vi "2photocell+ledcontrol+sum_cal.vi"() -> ()   [LabVIEW 2016]
uses:
  <vilib>/LabVIEW Interface for Arduino/LabVIEW Interface for Arduino.lvlib
  <vilib>/ptbypt/NI_PtbyPt.lvlib
panel:
  in  "stop":bool
  in  "Tab Control":enum32{"Page 1", "Page 2"}(tab)
  out "LUX":dbl
  out "Voltage":dbl(knob) scale=0.0..5.0
  out "Filtered x":dbl format="%0.2f"
  in  "br_coef":dbl
  in  "thrs low":i32=1
  in  "thrs high":i32=4
  in  "Slide 3":dbl(slide) min=0.0 max=255.0 scale=0.0..255.0
  in  "Slide 2":dbl(slide) min=0.0 max=255.0 scale=0.0..255.0
  in  "Slide":dbl(slide) min=0.0 max=255.0 scale=0.0..255.0
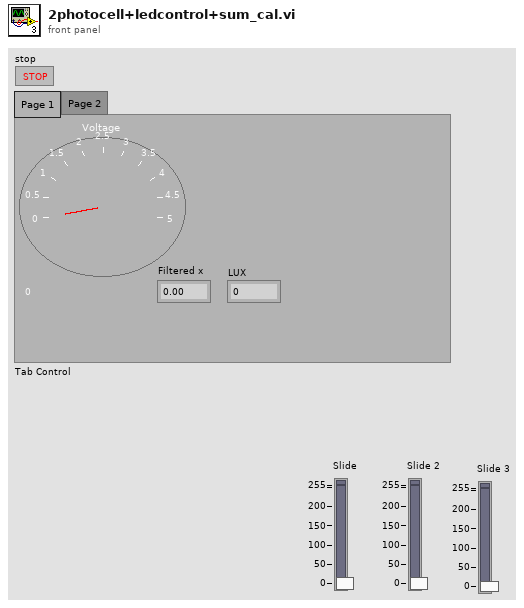
[diagram p1: front panel]
types:
  T1 = typedef "LabVIEW Interface for Arduino.lvlib/Arduino Resource.ctl" = cluster{"VISA resource":refnum<visa-resource-name>, "Board Type":T2, "Connection Type":enum8{"USB / Serial"}, "Bytes Per Packet (15)":u8}
  T2 = typedef "LabVIEW Interface for Arduino.lvlib/Board Type.ctl" = enum16{"Uno", "Dimuelanove w/Atmega 328", "Mega 2560"}
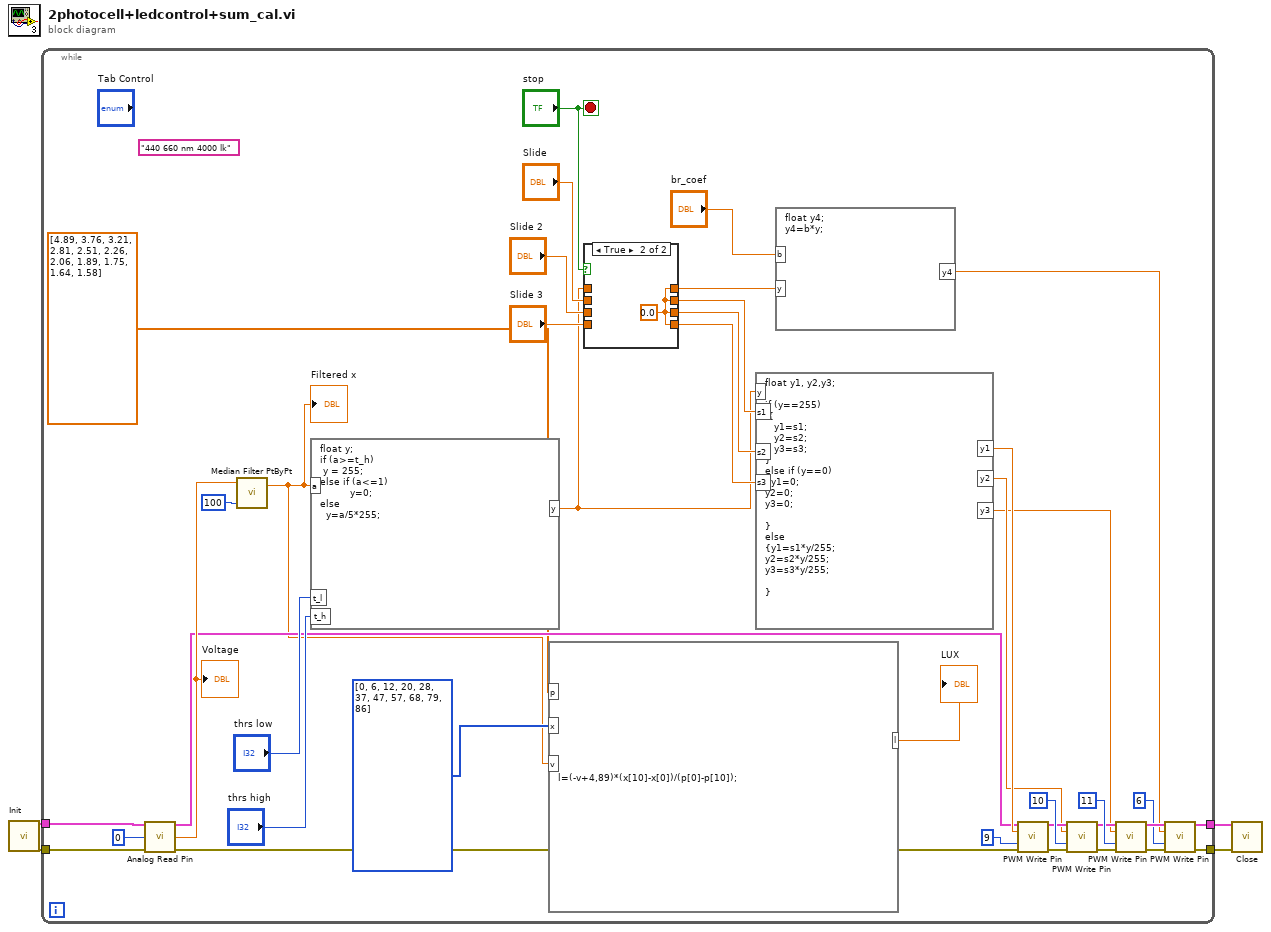
[diagram p0: block diagram]
diagram:
  n1 = call <vilib>:"Init.vi"() -> ("Arduino Resource"=w3:T1, "error out"=w4:errorcluster)  [unwired: 18 in]
  n2 = while {
    tunnel: w4 -> [w42]
    tunnel: w3 -> [w40]
    tunnel: [w18] -> w2
    tunnel: [w17] -> w1
    stop <- "stop" stop-if-true
    (unwired) "440 660 nm 4000 lk"
    n3 = call <vilib>:"Analog Read Pin.vi"("Arduino Resource"=w40, "Analog Input Pin (0)"=u8 0, "error in"=w42) -> ("Arduino Resource"=w10:T1, "Voltage"=w39:dbl, "error out"=w9:errorcluster)  [unwired: 10 in]
    "Voltage" <- w39
    n4 = call <vilib>:"Median Filter PtByPt.vi"("rank"=100, "x"=w39) -> ("Filtered x"=w6:dbl)  [unwired: 2 in, 1 out]
    "Filtered x" <- w6
    n5 = formula code="float y;\nif (a>=t_h)\n y = 255;\nelse if (a<=1)\n          y=0;\nelse\n  y=a/5*255;"("a"=w6, "t_l"="thrs low", "t_h"="thrs high") -> ("y"=w14:dbl)
    n6 = formula code="l=(-v+4,89)*(x[10]-x[0])/(p[0]-p[10]);"("x"=i32[] [0, 6, 12, 20, 28, 37, 47, 57, 68, 79, 86], "v"=w6, "p"=dbl[] [4.89, 3.76, 3.21, 2.81, 2.51, 2.26, 2.06, 1.89, 1.75, 1.64, 1.58]) -> ("l"=→"LUX":dbl)
    n7 = case shown="True" "stop" {
      tunnel: "Slide 2" -> [w47 _]
      tunnel: [w47 w48] -> w24
      tunnel: "Slide 3" -> [w46 _]
      tunnel: [w46 w48] -> w23
      tunnel: "Slide" -> [w45 _]
      tunnel: [w45 w48] -> w25
      tunnel: w14 -> [w44 _]
      tunnel: [w44 w48] -> w12
      frame False {
      }
      frame True {
        w48 = 0.0 ("Slide 2")
      }
    }
    n8 = formula code="float y1, y2,y3;\n\nif (y==255)\n {\n   y1=s1;\n   y2=s2;\n   y3=s3;\n}\nelse if (y==0)\n{y1=0;\ny2=0;\ny3=0;\n\n}\nelse \n{y1=s1*y/255;\ny2=s2*y/255;\ny3=s3*y/255;\n\n}"("s1"=w25, "s2"=w24, "s3"=w23, "y"=w14) -> ("y1"=w22:dbl, "y2"=w21:dbl, "y3"=w20:dbl)
    n9 = formula code="float y4;\ny4=b*y;"("b"="br_coef", "y"=w12) -> ("y4"=w11:dbl)
    n10 = call <vilib>:"PWM Write Pin.vi"("Arduino Resource"=w10, "Duty Cycle (0 - 255)"=w22, "PWM Pin (3)"=u8 9, "error in"=w9) -> ("Arduino Resource"=w31:T1, "error out"=w27:errorcluster)  [unwired: 10 in]
    n11 = call <vilib>:"PWM Write Pin.vi"("Arduino Resource"=w31, "Duty Cycle (0 - 255)"=w21, "PWM Pin (3)"=u8 10, "error in"=w27) -> ("Arduino Resource"=w30:T1, "error out"=w26:errorcluster)  [unwired: 10 in]
    n12 = call <vilib>:"PWM Write Pin.vi"("Arduino Resource"=w30, "Duty Cycle (0 - 255)"=w20, "PWM Pin (3)"=u8 11, "error in"=w26) -> ("Arduino Resource"=w19:T1, "error out"=w16:errorcluster)  [unwired: 10 in]
    n13 = call <vilib>:"PWM Write Pin.vi"("Arduino Resource"=w19, "Duty Cycle (0 - 255)"=w11, "PWM Pin (3)"=u8 6, "error in"=w16) -> ("Arduino Resource"=w18:T1, "error out"=w17:errorcluster)  [unwired: 10 in]
  }
  n14 = call <vilib>:"Close.vi"("Arduino Resource"=w2, "error in"=w1) -> ()  [unwired: 13 in, 1 out]
